vi "PWM Utility.vi"(9 "Break":bool, 10 "Enum":enum16{"3rd", "2nd", "1st", "N", "R"}(ring)=enum."R", 11 "GAS":bool) -> (2 "Red Lights":bool, 3 "PWM Width":dbl)   [LabVIEW 2015]
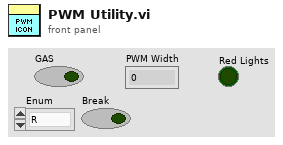
[diagram p1: front panel]
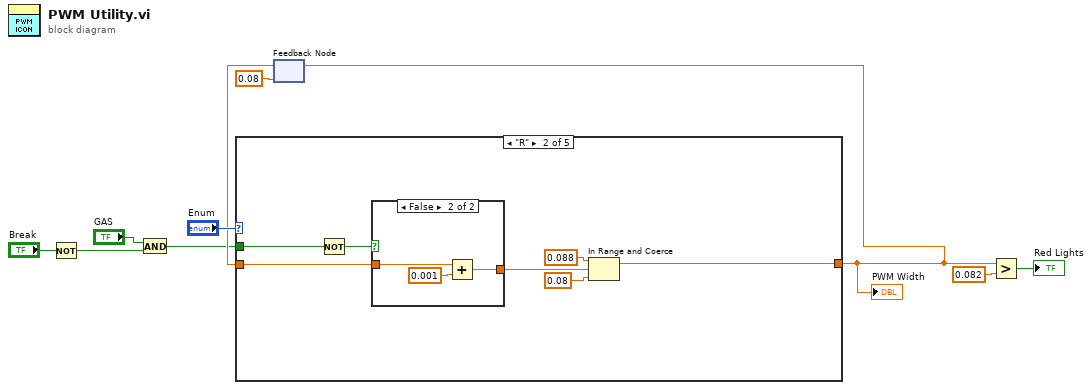
[diagram p0: block diagram]
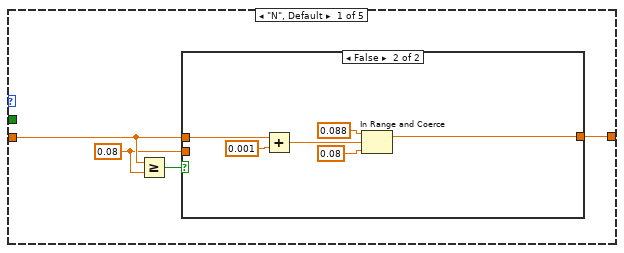
[diagram p2: hidden frame]
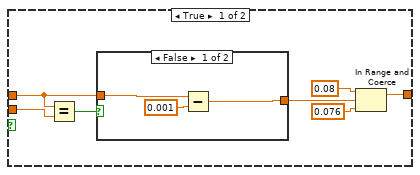
[diagram p3: hidden frame]
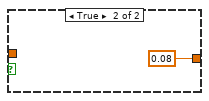
[diagram p4: hidden frame]
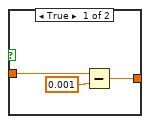
[diagram p5: hidden frame]
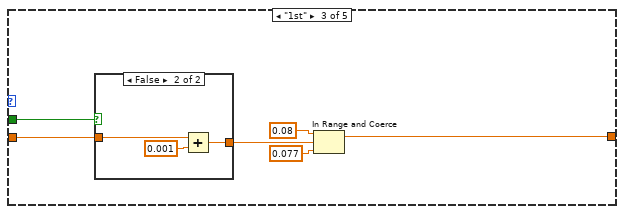
[diagram p6: hidden frame]
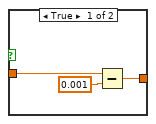
[diagram p7: hidden frame]
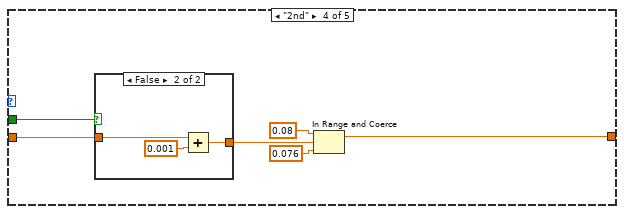
[diagram p8: hidden frame]
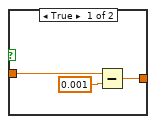
[diagram p9: hidden frame]
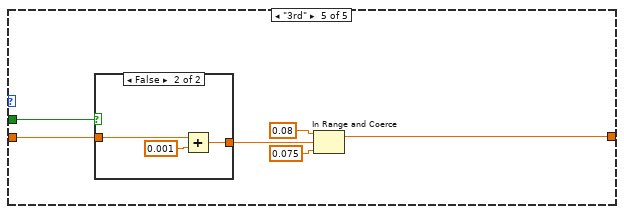
[diagram p10: hidden frame]
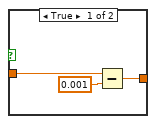
[diagram p11: hidden frame]
diagram:
  n1 = Not(x="Break") -> (.not. x?=w2:bool)
  n2 = And(x="GAS", y=w2) -> (x .and. y?=w1:bool)
  n3 = feedback #1(0.08) -> (w5:dbl)
  n4 = case shown="\"R\"" "Enum" {
    tunnel: w5 -> [w14 w35 w47 w59 w70]
    tunnel: [w12 w36 w48 w60 w72] -> w9
    tunnel: w1 -> [_ w33 w45 w58 w71]
    frame "N", Default {
      w11 = 0.08 ("y")
      n5 = Greater Or Equal?(x=w14, y=w11) -> (x >= y?=w13:bool)
      n6 = case shown="False" w13 {
        tunnel: w14 -> [w16 w28]
        tunnel: [w19 w29] -> w12
        tunnel: w11 -> [w17 _]
        frame True {
          n7 = Equal?(x=w16, y=w17) -> (x = y?=w18:bool)
          n8 = case shown="False" w18 {
            tunnel: w16 -> [w23 _]
            tunnel: [w22 0.08] -> w15
            frame False {
              n9 = Subtract(x=w23, y=0.001) -> (x-y=w22:dbl)
            }
            frame True {
            }
          }
          n10 = In Range and Coerce(upper limit=0.08, x=w15, lower limit=0.076) -> (coerced(x)=w19:dbl)  [unwired: 1 out]
        }
        frame False {
          n11 = Add(x=w28, y=0.001) -> (x+y=w27:dbl)
          n12 = In Range and Coerce(upper limit=0.088, x=w27, lower limit=0.08) -> (coerced(x)=w29:dbl)  [unwired: 1 out]
        }
      }
    }
    frame "R" {
      n13 = Not(x=w33) -> (.not. x?=w32:bool)
      n14 = case shown="False" w32 {
        tunnel: w35 -> [w41 w44]
        tunnel: [w40 w43] -> w34
        frame True {
          n15 = Subtract(x=w41, y=0.001) -> (x-y=w40:dbl)
        }
        frame False {
          n16 = Add(x=w44, y=0.001) -> (x+y=w43:dbl)
        }
      }
      n17 = In Range and Coerce(upper limit=0.088, x=w34, lower limit=0.08) -> (coerced(x)=w36:dbl)  [unwired: 1 out]
    }
    frame "1st" {
      n18 = case shown="False" w45 {
        tunnel: w47 -> [w53 w56]
        tunnel: [w52 w55] -> w46
        frame True {
          n19 = Subtract(x=w53, y=0.001) -> (x-y=w52:dbl)
        }
        frame False {
          n20 = Add(x=w56, y=0.001) -> (x+y=w55:dbl)
        }
      }
      n21 = In Range and Coerce(upper limit=0.08, x=w46, lower limit=0.077) -> (coerced(x)=w48:dbl)  [unwired: 1 out]
    }
    frame "2nd" {
      n22 = case shown="False" w58 {
        tunnel: w59 -> [w65 w68]
        tunnel: [w64 w67] -> w57
        frame True {
          n23 = Subtract(x=w65, y=0.001) -> (x-y=w64:dbl)
        }
        frame False {
          n24 = Add(x=w68, y=0.001) -> (x+y=w67:dbl)
        }
      }
      n25 = In Range and Coerce(upper limit=0.08, x=w57, lower limit=0.076) -> (coerced(x)=w60:dbl)  [unwired: 1 out]
    }
    frame "3rd" {
      n26 = case shown="False" w71 {
        tunnel: w70 -> [w77 w80]
        tunnel: [w76 w79] -> w69
        frame True {
          n27 = Subtract(x=w77, y=0.001) -> (x-y=w76:dbl)
        }
        frame False {
          n28 = Add(x=w80, y=0.001) -> (x+y=w79:dbl)
        }
      }
      n29 = In Range and Coerce(upper limit=0.08, x=w69, lower limit=0.075) -> (coerced(x)=w72:dbl)  [unwired: 1 out]
    }
  }
  "PWM Width" <- w9
  n30 = feedback-in #1(w9) -> ()
  n31 = Greater?(x=w9, y=0.082) -> (0:→"Red Lights":bool)
